vi "Application Configuration Path.vi"(11 "Application":T1) -> (3 "appended path":path)   [LabVIEW 2019, in "FP-TC-Shared.lvclass"]
uses:
  FP-TC-Shared.lvclass
  typedefs/Application Type--Enum.ctl
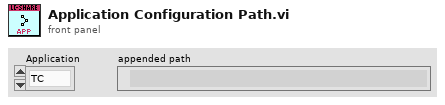
[diagram p1: front panel]
types:
  T1 = typedef "FP-TC-Shared.lvclass/Application Type--Enum.ctl" = enum16{"TC", "FP"}
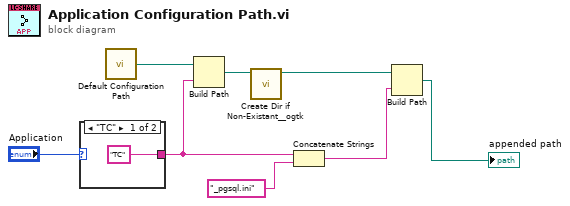
[diagram p0: block diagram]
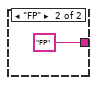
[diagram p2: hidden frame]
diagram:
  n1 = case shown="\"TC\"" "Application" {
    tunnel: ["TC" ("name or relative path") "FP" ("name or relative path")] -> w3
    frame "TC" {
    }
    frame "FP" {
    }
  }
  n2 = call "Default Configuration Path.vi"() -> ("base path"=w7:path)
  n3 = Build Path(base path=w7, name or relative path=w3) -> (appended path=w5:path)
  n4 = call <userlib>:"Create Dir if Non-Existant__ogtk.vi"("Directory Path"=w5) -> ("dup Directory Path"=w4:path)  [unwired: 8 in, 2 out]
  n5 = Concatenate Strings(w3, "_pgsql.ini" ("name or relative path")) -> (w1:string)
  n6 = Build Path(base path=w4, name or relative path=w1) -> (appended path=→"appended path":path)
